vi "DC Motor.vi"() -> ()   [LabVIEW 2017]
uses:
  DCMotor Controls.ctl
  <vilib>/DAQmx/read.llb/DAQmx Read (Counter DBL 1Chan 1Samp).vi
  <vilib>/DAQmx/create/channels.llb/DAQmx Create Channel (CO-Pulse Generation-Frequency).vi
  <vilib>/DAQmx/configure/timing.llb/DAQmx Timing (Implicit).vi
  <vilib>/DAQmx/create/channels.llb/DAQmx Create Channel (CI-Position-Angular Encoder).vi
  <vilib>/DAQmx/miscellaneous.llb/DAQmx Fill In Error Info.vi
  <resource>/objmgr/daqmx.rc
panel:
  in  "Encorder Counter 2":tag
  in  "A Input Terminal":tag
  in  "B Input Terminal":tag
  out "RPM":dbl
  out "Position (degrees)":dbl format="%0.2f"
  out "Current State":T1=enum."Stop"
  in  "Desired RPM":dbl=1000.0
  in  "Stop Program":bool
  in  "CO.Pulse.Term 2":tag="/Dev2/PFI1"
  in  "CO.Pulse.Term":tag="/Dev2/PFI0"
  in  "counter 2":tag="Dev2/ctr1"
  in  "counter":tag="Dev2/ctr0"
  in  "Speed":dbl(knob)=2.0 min=-49.0 max=2.0 step=1.0 scale=-49.0..2.0
  in  "Forward":bool
  in  "Start/Stop Motor":bool
  # "Board Counters"
  # "Motor Controls"
  # "Encoder Readings"
  # "Encoder Input Terminals"
  # "Pulse Output Terminals"
  # "Reverse"
  # "Fast"
  # "Slow"
  # "Vcc2 should be 9V - not 24V!"
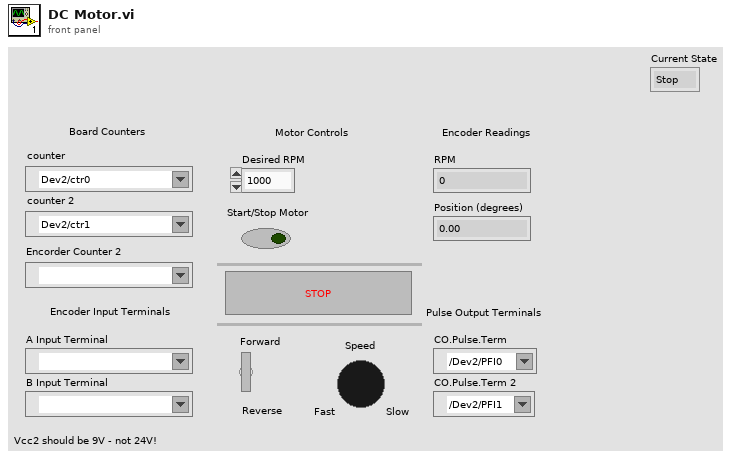
[diagram p1: front panel]
types:
  T1 = typedef "DCMotor Controls.ctl" = enum16{"Wait for UI", "Update", "Stop"}
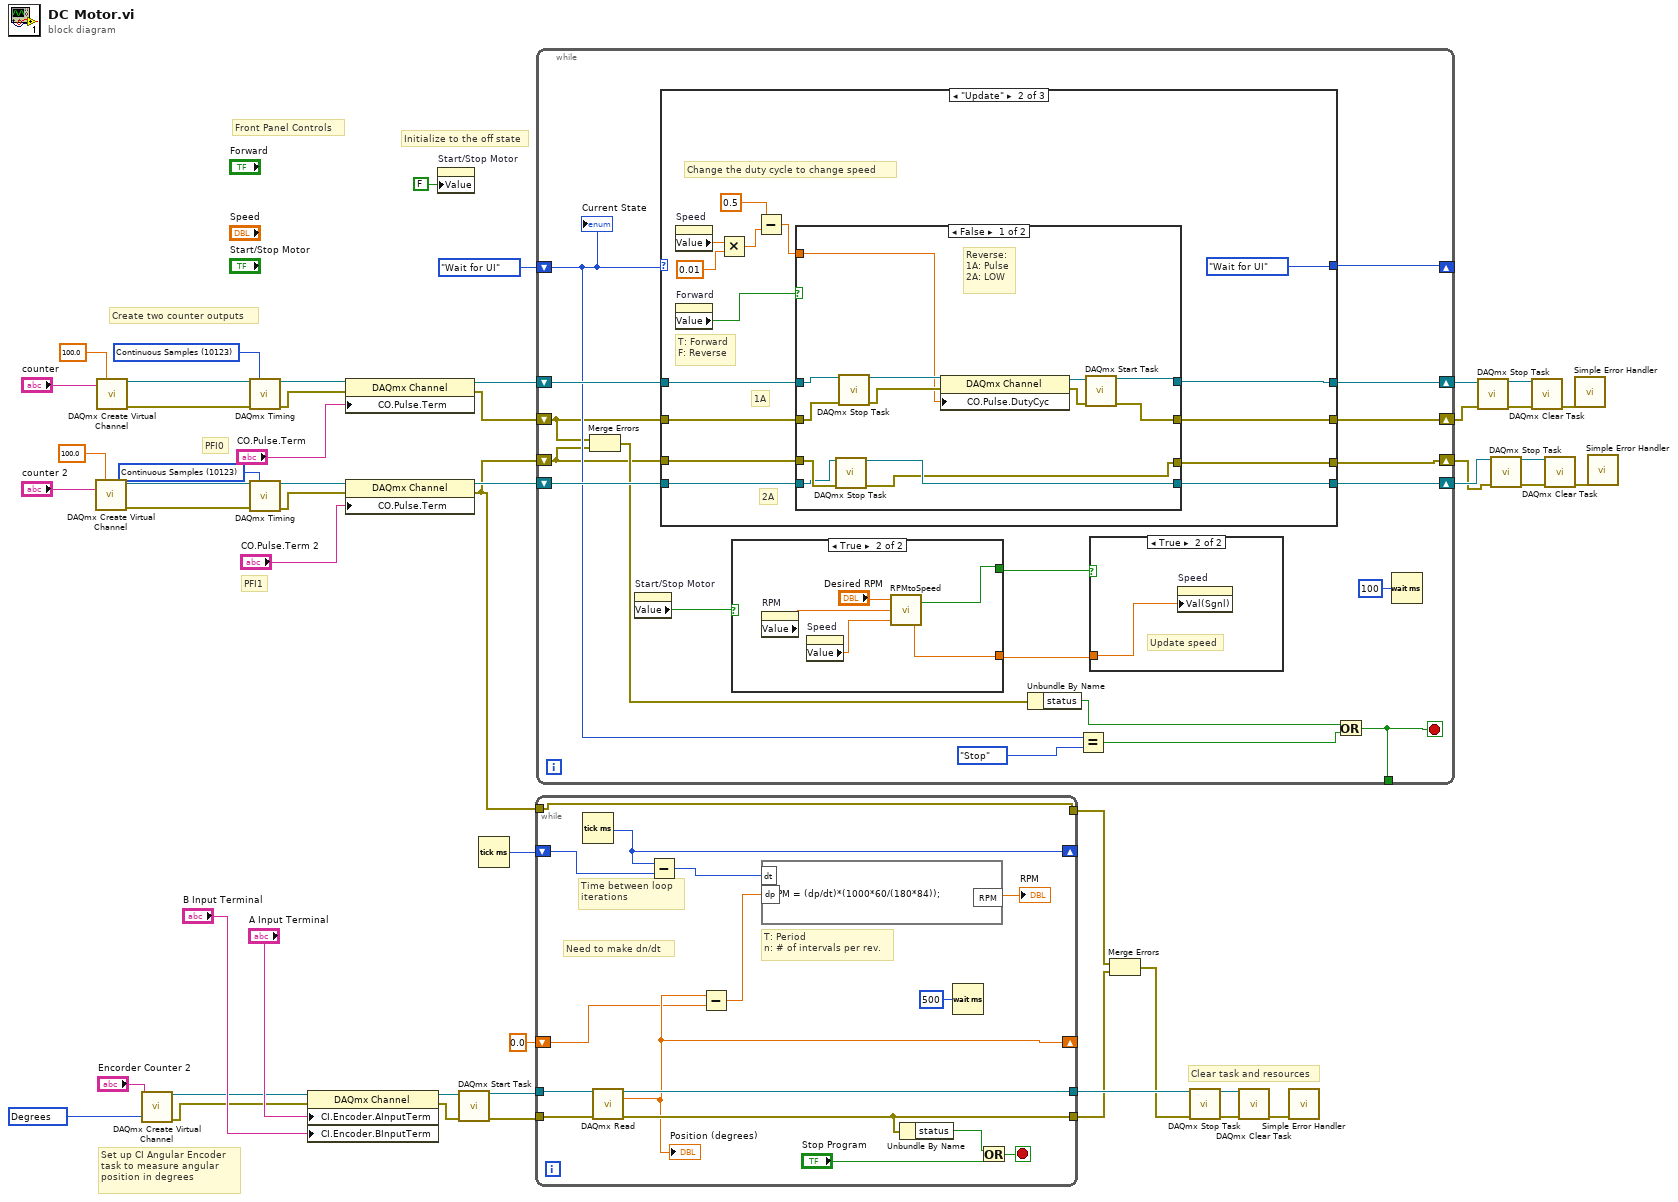
[diagram p0: block diagram]
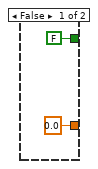
[diagram p2: hidden frame]
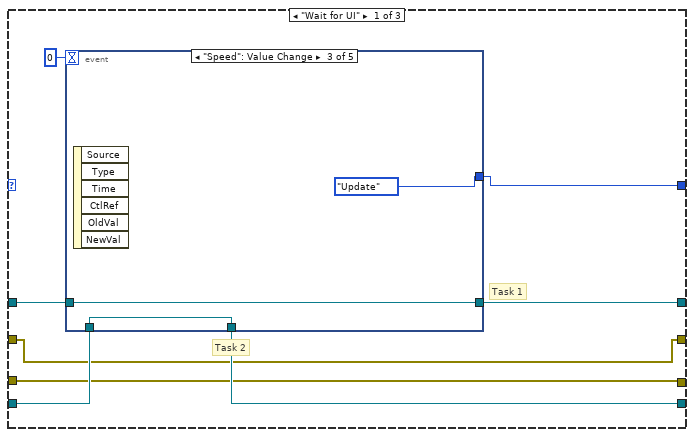
[diagram p4: hidden frame]
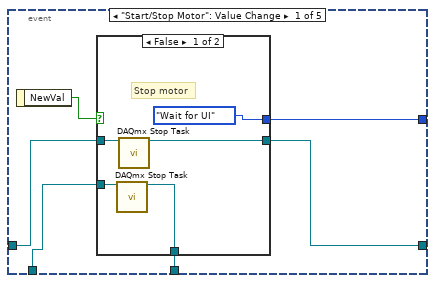
[diagram p5: hidden frame]
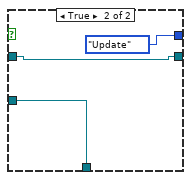
[diagram p6: hidden frame]
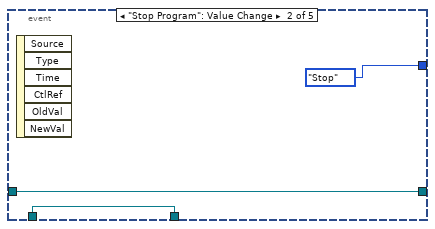
[diagram p7: hidden frame]
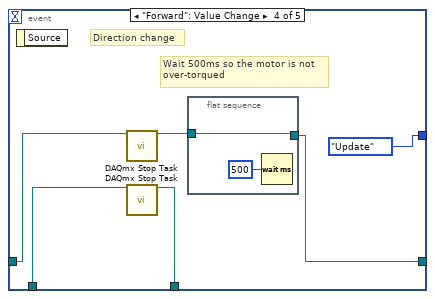
[diagram p8: hidden frame]
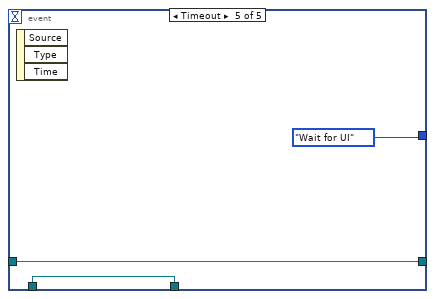
[diagram p9: hidden frame]
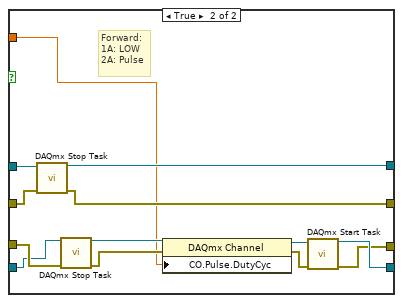
[diagram p10: hidden frame]
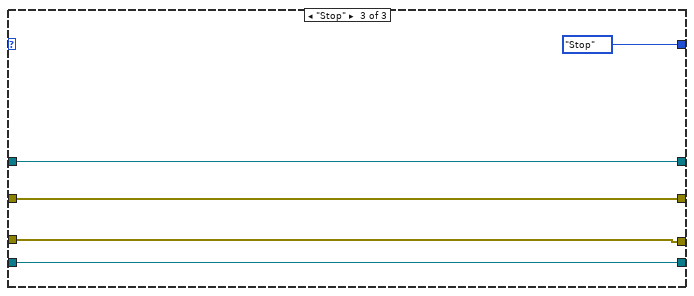
[diagram p11: hidden frame]
diagram:
  w5 = 10146 items=["Degrees"=10146, "Radians"=10273, "Ticks"=10304, "From Custom Scale"=10065] ("units")
  w32 = 10123 items=["Finite Samples"=10178, "Continuous Samples"=10123, "Hardware Timed Single Point"=12522] ("sample mode")
  w33 = 10123 items=["Finite Samples"=10178, "Continuous Samples"=10123, "Hardware Timed Single Point"=12522] ("sample mode")
  # "Clear task and resources"
  # "Set up CI Angular Encoder\ntask to measure angular\nposition in degrees"
  # "PFI1"
  # "PFI0"
  # "Initialize to the off state"
  # "Front Panel Controls"
  # "Create two counter outputs"
  n1 = call-poly <vilib>:"DAQmx Create Virtual Channel.vi"("frequency"=100.0, "counter"="counter 2") -> ("task out"=w50:refnum<k21>, "error out"=w40:errorcluster)  [unwired: 12 in]
  n2 = call-poly <vilib>:"DAQmx Create Virtual Channel.vi"("frequency"=100.0, "counter"="counter") -> ("task out"=w51:refnum<k21>, "error out"=w42:errorcluster)  [unwired: 12 in]
  n3 = call-poly <vilib>:"DAQmx Create Virtual Channel.vi"("counter"="Encorder Counter 2", "units"=w5) -> ("task out"=w7:refnum<k21>, "error out"=w8:errorcluster)  [unwired: 12 in]
  n4 = call-poly <vilib>:"DAQmx Timing.vi"("task/channels in"=w51, "sample mode"=w33, "error in"=w42) -> ("task out"=w49:refnum<k21>, "error out"=w41:errorcluster)  [unwired: 11 in]
  n5 = call-poly <vilib>:"DAQmx Timing.vi"("task/channels in"=w50, "sample mode"=w32, "error in"=w40) -> ("task out"=w45:refnum<k21>, "error out"=w39:errorcluster)  [unwired: 11 in]
  n6 = property class="DAQmx Channel"(reference=w7, error in=w8, "CI.Encoder.AInputTerm"="A Input Terminal", "CI.Encoder.BInputTerm"="B Input Terminal") -> (reference out=w11:refnum<k21>, error out=w12:errorcluster)
  n7 = property class="DAQmx Channel"(reference=w49, error in=w41, "CO.Pulse.Term"="CO.Pulse.Term") -> (reference out=w38:refnum<k21>, error out=w34:errorcluster)
  n8 = property class="DAQmx Channel"(reference=w45, error in=w39, "CO.Pulse.Term"="CO.Pulse.Term 2") -> (reference out=w37:refnum<k21>, error out=w4:errorcluster)
  n9 = property on="Start/Stop Motor" class="Bool (strict)"("Value"=FALSE ("Start/Stop Motor")) -> ()  [unwired: 2 in, 2 out]
  n10 = call <vilib>:"DAQmx Start Task.vi"("task/channels in"=w11, "error in"=w12) -> ("task out"=w13:refnum<k21>, "error out"=w14:errorcluster)  [unwired: 12 in]
  n11 = Tick Count (ms)() -> (millisecond timer value=w19:u32)
  n12 = while {
    tunnel: w13 -> [w67]
    tunnel: w14 -> [w66]
    tunnel: [w63] -> w2
    tunnel: [w64] -> w15
    shift-right: [w60] -> _
    shift-left: w19 -> [w61]
    shift-right: [w57] -> _
    shift-left: 0.0 ("data") -> [w56]
    tunnel: [w53] -> w3
    tunnel: w4 -> [w53]
    stop <- w65 stop-if-true
    # "Need to make dn/dt"
    # "Time between loop\niterations"
    # "T: Period\nn: # of intervals per rev."
    n13 = Tick Count (ms)() -> (millisecond timer value=w60:u32)
    n14 = call-poly <vilib>:"DAQmx Read.vi"("task/channels in"=w67, "error in"=w66) -> ("task out"=w64:refnum<k21>, "data"=w57:dbl, "error out"=w63:errorcluster)  [unwired: 11 in]
    "Position (degrees)" <- w57
    n15 = Subtract(x=w60, y=w61) -> (x-y=w59:u32)
    n16 = Subtract(x=w57, y=w56) -> (x-y=w55:dbl)
    n17 = formula code="RPM = (dp/dt)*(1000*60/(180*84));"("dt"=w59, "dp"=w55) -> ("RPM"=→"RPM":dbl)
    n18 = Unbundle By Name(w63) -> ("status"=w62:bool)
    n19 = Wait (ms)(milliseconds to wait=u32 500) -> ()  [unwired: 1 out]
    n20 = Or(x=w62, y="Stop Program") -> (x .or. y?=w65:bool)
  }
  n21 = while {
    shift-right: [w80] -> w31
    shift-left: w38 -> [w86]
    shift-right: [w79] -> w23
    shift-left: w37 -> [w85]
    shift-right: [w81] -> _
    shift-left: DCMotor_Controls."Wait for UI" -> [w83]
    shift-right: [w75] -> w30
    shift-left: w34 -> [w77]
    shift-right: [w74] -> w22
    shift-left: w4 -> [w76]
    tunnel: [w72] -> _
    stop <- w72 stop-if-true
    n22 = Merge Errors(w77, w76) -> (w78:errorcluster)
    n23 = property on="Start/Stop Motor" class="Bool (strict)"() -> ("Value"=w69:bool)  [unwired: 2 in, 2 out]
    n24 = case shown="\"Update\"" w83 {
      tunnel: w86 -> [w102 w145 w178]
      tunnel: w85 -> [w100 w144 w175]
      tunnel: [w98 DCMotor_Controls."Wait for UI" DCMotor_Controls."Stop"] -> w81
      tunnel: [w101 w141 w178] -> w80
      tunnel: [w99 w139 w175] -> w79
      tunnel: w77 -> [w97 w143 w177]
      tunnel: w76 -> [w96 w142 w176]
      tunnel: [w97 w140 w177] -> w75
      tunnel: [w96 w138 w176] -> w74
      frame "Wait for UI" {
        # "Task 2"
        # "Task 1"
        n25 = event shown="[2] \"Speed\": Value Change" {
          selector: _ -> [_ _ _ _ _]
          dyn-events: _ -> [_ _ _ _ _]
          timeout: 0 -> [_ _ _ _ _]
          tunnel: w102 -> [w106 w119 w122 w128 w131]
          tunnel: [w104 w119 w122 w126 w131] -> w101
          tunnel: w100 -> [w105 w118 w121 w125 w132]
          tunnel: [w103 w118 w121 w124 w132] -> w99
          tunnel: [w107 DCMotor_Controls."Stop" DCMotor_Controls."Update" DCMotor_Controls."Update" DCMotor_Controls."Wait for UI"] -> w98
          event "Start/Stop Motor": Value Change {
            n26 = event-data() -> ("NewVal"=w108:bool)  [unwired: 1 in]
            n27 = case shown="False" w108 {
              tunnel: [DCMotor_Controls."Wait for UI" DCMotor_Controls."Update"] -> w107
              tunnel: w106 -> [w113 w115]
              tunnel: w105 -> [w112 w114]
              tunnel: [w111 w115] -> w104
              tunnel: [w110 w114] -> w103
              frame False {
                # "Stop motor"
                n28 = call <vilib>:"DAQmx Stop Task.vi"("task/channels in"=w112) -> ("task out"=w110:refnum<k21>)  [unwired: 13 in, 1 out]
                n29 = call <vilib>:"DAQmx Stop Task.vi"("task/channels in"=w113) -> ("task out"=w111:refnum<k21>)  [unwired: 13 in, 1 out]
              }
              frame True {
              }
            }
          }
          event "Stop Program": Value Change {
            n30 = event-data() -> ()  [unwired: 1 in, 6 out]
          }
          event "Speed": Value Change {
            n31 = event-data() -> ()  [unwired: 1 in, 6 out]
          }
          event "Forward": Value Change {
            # "Wait 500ms so the motor is not\nover-torqued"
            # "Direction change"
            n32 = event-data() -> ()  [unwired: 1 in, 1 out]
            n33 = call <vilib>:"DAQmx Stop Task.vi"("task/channels in"=w128) -> ("task out"=w127:refnum<k21>)  [unwired: 13 in, 1 out]
            n34 = call <vilib>:"DAQmx Stop Task.vi"("task/channels in"=w125) -> ("task out"=w124:refnum<k21>)  [unwired: 13 in, 1 out]
            n35 = flat-sequence {
              tunnel: w127 -> [w129]
              tunnel: [w129] -> w126
              frame #0 {
                n36 = Wait (ms)(milliseconds to wait=u32 500) -> ()  [unwired: 1 out]
              }
            }
          }
          event Timeout {
            n37 = event-data() -> ()  [unwired: 1 in, 3 out]
          }
        }
      }
      frame "Update" {
        # "Change the duty cycle to change speed"
        # "2A"
        # "1A"
        # "T: Forward\nF: Reverse"
        n38 = property on="Speed" class="Knob (strict)"() -> ("Value"=w148:dbl)  [unwired: 2 in, 2 out]
        n39 = property on="Forward" class="Bool (strict)"() -> ("Value"=w146:bool)  [unwired: 2 in, 2 out]
        n40 = Multiply(x=w148, y=0.01) -> (x*y=w134:dbl)
        n41 = Subtract(x=0.5, y=w134) -> (x-y=w135:dbl)
        n42 = case shown="False" w146 {
          tunnel: w145 -> [w157 w174]
          tunnel: w144 -> [w152 w169]
          tunnel: w143 -> [w156 w173]
          tunnel: w142 -> [w153 w170]
          tunnel: [w155 w166] -> w141
          tunnel: [w154 w165] -> w140
          tunnel: [w151 w164] -> w139
          tunnel: [w150 w163] -> w138
          tunnel: w135 -> [w149 w162]
          frame False {
            # "Reverse:\n1A: Pulse\n2A: LOW"
            n43 = call <vilib>:"DAQmx Stop Task.vi"("task/channels in"=w152, "error in"=w153) -> ("task out"=w151:refnum<k21>, "error out"=w150:errorcluster)  [unwired: 12 in]
            n44 = call <vilib>:"DAQmx Stop Task.vi"("task/channels in"=w157, "error in"=w156) -> ("task out"=w159:refnum<k21>, "error out"=w158:errorcluster)  [unwired: 12 in]
            n45 = property class="DAQmx Channel"(reference=w159, error in=w158, "CO.Pulse.DutyCyc"=w149) -> (reference out=w161:refnum<k21>, error out=w160:errorcluster)
            n46 = call <vilib>:"DAQmx Start Task.vi"("task/channels in"=w161, "error in"=w160) -> ("task out"=w155:refnum<k21>, "error out"=w154:errorcluster)  [unwired: 12 in]
          }
          frame True {
            # "Forward:\n1A: LOW\n2A: Pulse"
            n47 = call <vilib>:"DAQmx Stop Task.vi"("task/channels in"=w174, "error in"=w173) -> ("task out"=w166:refnum<k21>, "error out"=w165:errorcluster)  [unwired: 12 in]
            n48 = call <vilib>:"DAQmx Stop Task.vi"("task/channels in"=w169, "error in"=w170) -> ("task out"=w168:refnum<k21>, "error out"=w167:errorcluster)  [unwired: 12 in]
            n49 = property class="DAQmx Channel"(reference=w168, error in=w167, "CO.Pulse.DutyCyc"=w162) -> (reference out=w172:refnum<k21>, error out=w171:errorcluster)
            n50 = call <vilib>:"DAQmx Start Task.vi"("task/channels in"=w172, "error in"=w171) -> ("task out"=w164:refnum<k21>, "error out"=w163:errorcluster)  [unwired: 12 in]
          }
        }
      }
      frame "Stop" {
      }
    }
    n51 = case shown="True" w69 {
      tunnel: [0.0 ("New Speed") w90] -> w71
      tunnel: [FALSE ("Update?") w89] -> w70
      frame False {
      }
      frame True {
        n52 = property on="RPM" class="DigNum (strict)"() -> ("Value"=w93:dbl)  [unwired: 2 in, 2 out]
        n53 = property on="Speed" class="Knob (strict)"() -> ("Value"=w91:dbl)  [unwired: 2 in, 2 out]
        n54 = call "RPMtoSpeed.vi"("Speed"=w91, "Measured RPM"=w93, "Desired RPM"="Desired RPM") -> ("New Speed"=w90:dbl, "Update?"=w89:bool)
      }
    }
    n55 = Unbundle By Name(w78) -> ("status"=w73:bool)
    n56 = Equal?(x=w83, y=DCMotor_Controls."Stop") -> (x = y?=w82:bool)
    n57 = case shown="True" w70 {
      tunnel: w71 -> [_ w94]
      frame False {
        # "Do nothing"
      }
      frame True {
        # "Update speed"
        n58 = property on="Speed" class="Knob (strict)"("Val(Sgnl)"=w94) -> ()  [unwired: 2 in, 2 out]
      }
    }
    n59 = Or(x=w73, y=w82) -> (x .or. y?=w72:bool)
    n60 = Wait (ms)(milliseconds to wait=u32 100) -> ()  [unwired: 1 out]
    "Current State" <- w83
  }
  n61 = Merge Errors(w3, w2) -> (w1:errorcluster)
  n62 = call <vilib>:"DAQmx Stop Task.vi"("task/channels in"=w15, "error in"=w1) -> ("task out"=w16:refnum<k21>, "error out"=w17:errorcluster)  [unwired: 12 in]
  n63 = call <vilib>:"DAQmx Clear Task.vi"("task in"=w16, "error in"=w17) -> ("error out"=w18:errorcluster)  [unwired: 13 in]
  n64 = call <vilib>:"Simple Error Handler.vi"("error in (no error)"=w18) -> ()  [unwired: 4 in, 5 out]
  n65 = call <vilib>:"DAQmx Stop Task.vi"("task/channels in"=w31, "error in"=w30) -> ("task out"=w29:refnum<k21>, "error out"=w28:errorcluster)  [unwired: 12 in]
  n66 = call <vilib>:"DAQmx Stop Task.vi"("task/channels in"=w23, "error in"=w22) -> ("task out"=w24:refnum<k21>, "error out"=w25:errorcluster)  [unwired: 12 in]
  n67 = call <vilib>:"DAQmx Clear Task.vi"("task in"=w29, "error in"=w28) -> ("error out"=w27:errorcluster)  [unwired: 13 in]
  n68 = call <vilib>:"DAQmx Clear Task.vi"("task in"=w24, "error in"=w25) -> ("error out"=w26:errorcluster)  [unwired: 13 in]
  n69 = call <vilib>:"Simple Error Handler.vi"("error in (no error)"=w27) -> ()  [unwired: 4 in, 5 out]
  n70 = call <vilib>:"Simple Error Handler.vi"("error in (no error)"=w26) -> ()  [unwired: 4 in, 5 out]
